vi "quality of life shit.vi"() -> ()   [LabVIEW 2021]
uses:
  <userlib>/Nanonis Prog Interface V5/Nanonis Prog Interface.lvlib
panel:
  in  "?":T1(tab)
  in  "Scan Frame":bool
  in  "Walk out":bool
  in  "Walk out Amplitude (V)":sgl=320.0
  in  "Walk out steps per set":u16=10
  in  "Number of sets of steps":i32=7
  in  "Stop approach":bool
  in  "Approach voltage":dbl=220.0
  in  "Approach":bool
  in  "Amplitude (V)":dbl=0.01
  in  "Frequency (Hz)":dbl=381.7
  in  "Set lockin \nparameters":bool
  in  "Make current \nbias start":bool
  in  "Mirror start":bool
  in  "Start voltage (V)":dbl
  in  "End voltage (V)":dbl
  in  "Set values":bool
  # "to Tip"
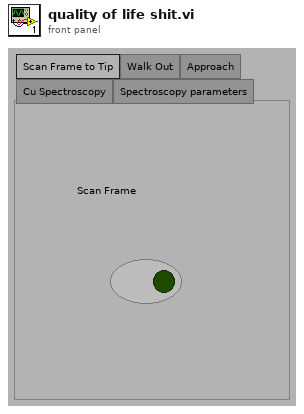
[diagram p1: front panel]
types:
  T1 = enum32{"Scan Frame to Tip", "Walk Out", "Approach", "Cu Spectroscopy", "Spectroscopy parameters"}
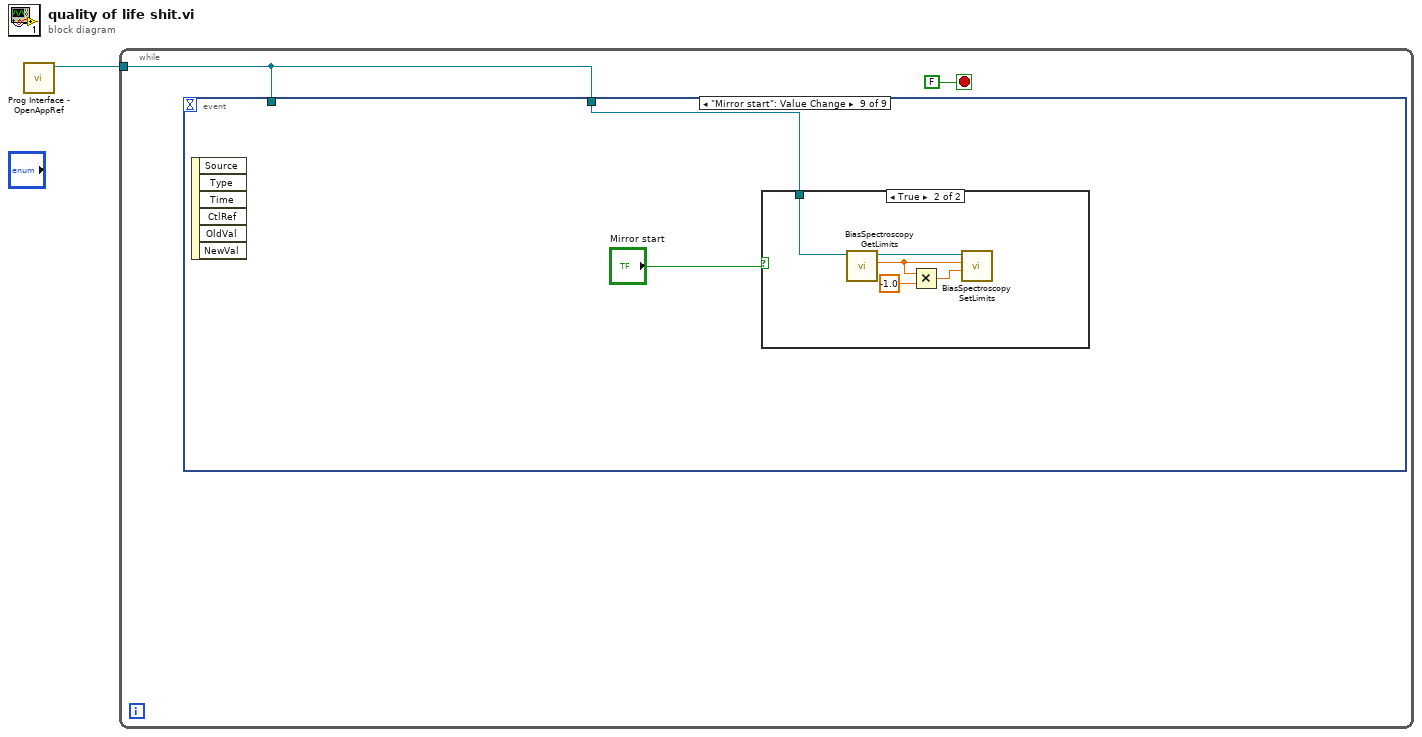
[diagram p0: block diagram]
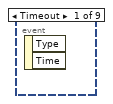
[diagram p2: hidden frame]
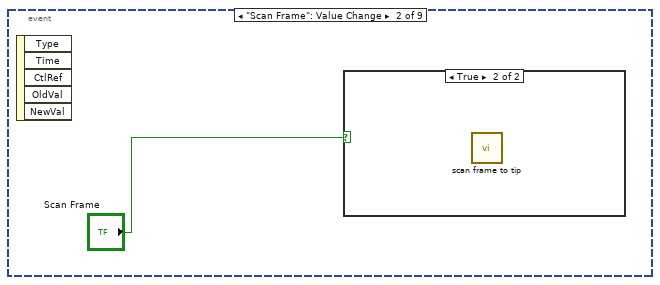
[diagram p3: hidden frame]
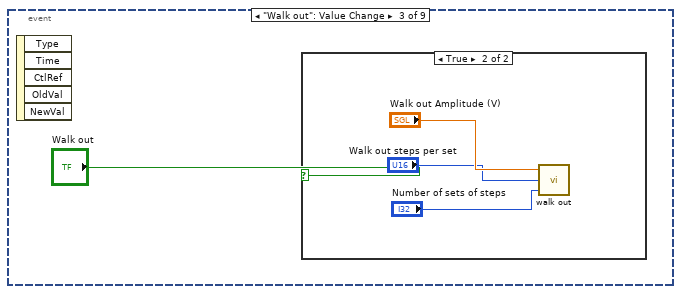
[diagram p5: hidden frame]
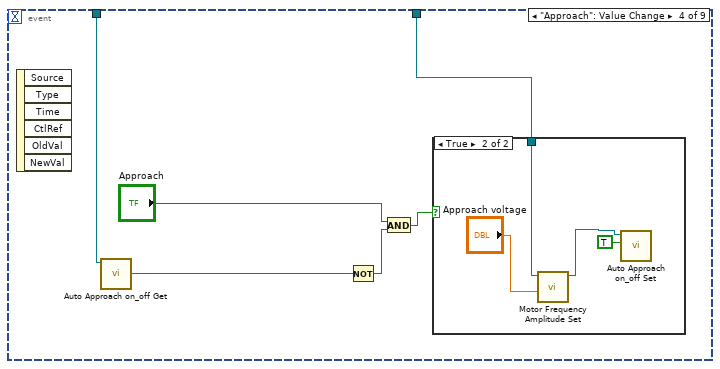
[diagram p7: hidden frame]
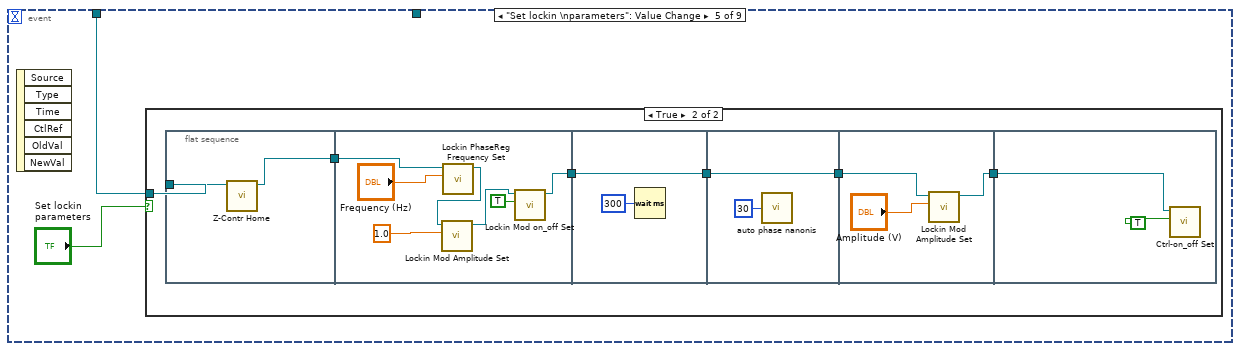
[diagram p9: hidden frame]
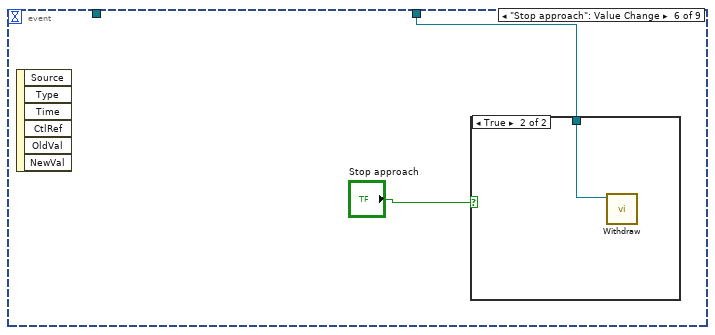
[diagram p11: hidden frame]
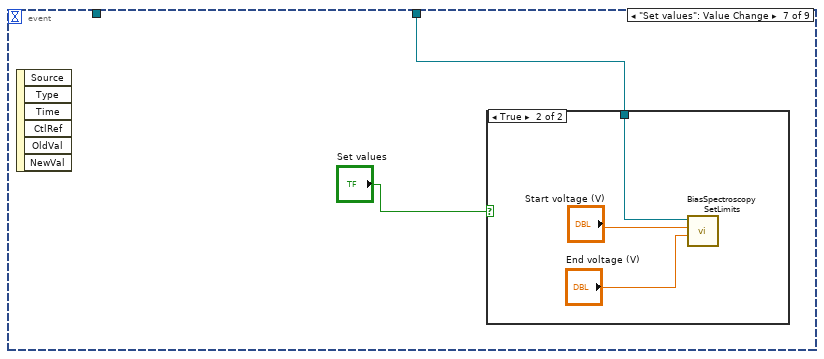
[diagram p13: hidden frame]
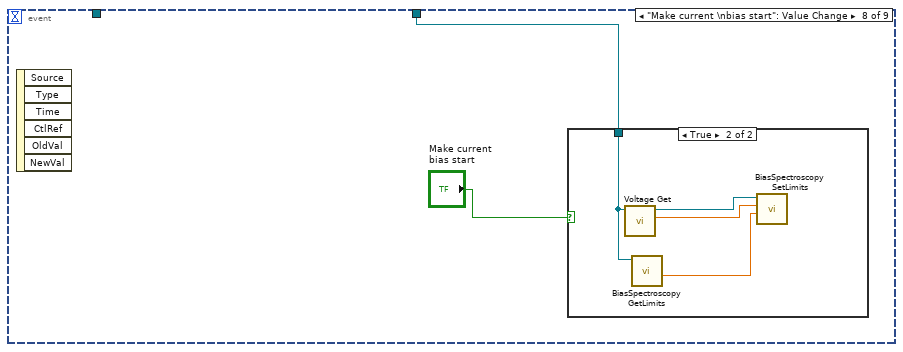
[diagram p15: hidden frame]
diagram:
  n1 = call <userlib>:"Prog Interface - OpenAppRef.vi"() -> ("Application reference"=w1:refnum<vi>)  [unwired: 6 in, 1 out]
  n2 = while {
    tunnel: w1 -> [w2]
    stop <- FALSE stop-if-true
    n3 = event shown="[8] \"Mirror start\": Value Change" {
      selector: _ -> [_ _ _ _ _ _ _ _ _]
      dyn-events: _ -> [_ _ _ _ _ _ _ _ _]
      timeout: _ -> [_ _ _ _ _ _ _ _ _]
      tunnel: w2 -> [_ _ _ w14 _ w45 w48 w53 w59]
      tunnel: w2 -> [_ _ _ w9 w19 _ _ _ _]
      event Timeout {
        n4 = event-data() -> ()  [unwired: 1 in, 2 out]
      }
      event "Scan Frame": Value Change {
        n5 = event-data() -> ()  [unwired: 1 in, 5 out]
        n6 = case shown="True" "Scan Frame" {
          frame False {
          }
          frame True {
            n7 = call "scan frame to tip.vi"() -> ()  [unwired: 12 in]
          }
        }
      }
      event "Walk out": Value Change {
        n8 = event-data() -> ()  [unwired: 1 in, 5 out]
        n9 = case shown="True" "Walk out" {
          frame False {
          }
          frame True {
            n10 = call "walk out.vi"("Number of sets of steps"="Number of sets of steps", "Walk out number steps"="Walk out steps per set", "Walk out Amplitude (V)"="Walk out Amplitude (V)") -> ()
          }
        }
      }
      event "Approach": Value Change {
        n11 = event-data() -> ()  [unwired: 1 in, 6 out]
        n12 = call <userlib>:"Auto Approach on_off Get.vi"("Application ref in"=w9) -> ("Auto approach on/off status"=w13:bool)  [unwired: 6 in, 2 out]
        n13 = Not(x=w13) -> (.not. x?=w11:bool)
        n14 = And(x="Approach", y=w11) -> (x .and. y?=w12:bool)
        n15 = case shown="True" w12 {
          tunnel: w14 -> [_ w16]
          frame False {
          }
          frame True {
            n16 = call <userlib>:"Motor Frequency Amplitude Set.vi"("Amplitude (V) (NaN=no change)"="Approach voltage", "Application ref in"=w16) -> ("Application ref out"=w15:refnum<vi>)  [unwired: 8 in, 1 out]
            n17 = call <userlib>:"Auto Approach on_off Set.vi"("Auto approach start/stop (F)"=TRUE, "Application ref in"=w15) -> ()  [unwired: 6 in, 2 out]
          }
        }
      }
      event "Set lockin \nparameters": Value Change {
        n18 = event-data() -> ()  [unwired: 1 in, 6 out]
        n19 = case shown="True" "Set lockin \nparameters" {
          tunnel: w19 -> [_ w26]
          frame False {
          }
          frame True {
            n20 = flat-sequence {
              tunnel: w26 -> [w28]
              tunnel: [w27] -> w25
              tunnel: w25 -> [w32]
              tunnel: [w29] -> w23
              tunnel: [w36] -> w24
              tunnel: w23 -> [w36]
              tunnel: [w38] -> w22
              tunnel: w24 -> [w38]
              tunnel: w22 -> [w41]
              tunnel: [w40] -> w21
              tunnel: w21 -> [w43]
              frame #0 {
                n21 = call <userlib>:"Z-Contr Home.vi"("Application ref in"=w28) -> ("Application ref out"=w27:refnum<vi>)  [unwired: 9 in, 1 out]
              }
              frame #1 {
                n22 = call <userlib>:"Lockin PhaseReg Frequency Set.vi"("Frequency (Hz)"="Frequency (Hz)", "Application ref in"=w32) -> ("Application ref out"=w31:refnum<vi>)  [unwired: 8 in, 1 out]
                n23 = call <userlib>:"Lockin Mod Amplitude Set.vi"("Amplitude (mod. signal unit)"=sgl 1.0, "Application ref in"=w31) -> ("Application ref out"=w30:refnum<vi>)  [unwired: 8 in, 1 out]
                n24 = call <userlib>:"Lockin Mod on_off Set.vi"("Lockin ON/OFF"=TRUE, "Application ref in"=w30) -> ("Application ref out"=w29:refnum<vi>)  [unwired: 8 in, 1 out]
              }
              frame #2 {
                n25 = Wait (ms)(milliseconds to wait=u32 300) -> ()  [unwired: 1 out]
              }
              frame #3 {
                n26 = call "auto phase nanonis.vi"("Num averages"=u32 30) -> ()
              }
              frame #4 {
                n27 = call <userlib>:"Lockin Mod Amplitude Set.vi"("Amplitude (mod. signal unit)"="Amplitude (V)", "Application ref in"=w41) -> ("Application ref out"=w40:refnum<vi>)  [unwired: 8 in, 1 out]
              }
              frame #5 {
                n28 = call <userlib>:"Ctrl-on_off Set.vi"("Z Controller ON/OFF"=TRUE, "Application ref in"=w43) -> ()  [unwired: 8 in, 2 out]
              }
            }
          }
        }
      }
      event "Stop approach": Value Change {
        n29 = event-data() -> ()  [unwired: 1 in, 6 out]
        n30 = case shown="True" "Stop approach" {
          tunnel: w45 -> [_ w47]
          frame False {
          }
          frame True {
            n31 = call <userlib>:"Withdraw.vi"("Application ref in"=w47) -> ()  [unwired: 9 in, 2 out]
          }
        }
      }
      event "Set values": Value Change {
        n32 = event-data() -> ()  [unwired: 1 in, 6 out]
        n33 = case shown="True" "Set values" {
          tunnel: w48 -> [_ w50]
          frame False {
          }
          frame True {
            n34 = call <userlib>:"BiasSpectroscopy SetLimits.vi"("End value (V)"="End voltage (V)", "Start value (V)"="Start voltage (V)", "Application ref in"=w50) -> ()  [unwired: 5 in, 2 out]
          }
        }
      }
      event "Make current \nbias start": Value Change {
        n35 = event-data() -> ()  [unwired: 1 in, 6 out]
        n36 = case shown="True" "Make current \nbias start" {
          tunnel: w53 -> [_ w55]
          frame False {
          }
          frame True {
            n37 = call <userlib>:"Voltage Get.vi"("Application ref in"=w55) -> ("Bias (V)"=w58:sgl, "Application ref out"=w57:refnum<vi>)  [unwired: 8 in, 1 out]
            n38 = call <userlib>:"BiasSpectroscopy GetLimits.vi"("Application ref in"=w55) -> ("End value (V)"=w56:sgl)  [unwired: 5 in, 3 out]
            n39 = call <userlib>:"BiasSpectroscopy SetLimits.vi"("End value (V)"=w56, "Start value (V)"=w58, "Application ref in"=w57) -> ()  [unwired: 5 in, 2 out]
          }
        }
      }
      event "Mirror start": Value Change {
        n40 = event-data() -> ()  [unwired: 1 in, 6 out]
        n41 = case shown="True" "Mirror start" {
          tunnel: w59 -> [_ w65]
          frame False {
          }
          frame True {
            n42 = call <userlib>:"BiasSpectroscopy GetLimits.vi"("Application ref in"=w65) -> ("Start value (V)"=w61:sgl, "Application ref out"=w64:refnum<vi>)  [unwired: 5 in, 2 out]
            n43 = Multiply(x=w61, y=-1.0) -> (x*y=w62:dbl)
            n44 = call <userlib>:"BiasSpectroscopy SetLimits.vi"("End value (V)"=w62, "Start value (V)"=w61, "Application ref in"=w64) -> ()  [unwired: 5 in, 2 out]
          }
        }
      }
    }
  }
